vi "TTLConnect.vi"(0 "port":u16, 1 "error in":errorcluster) -> (2 "context out":refnum<class "zmq_context.lvclass">, 3 "socket out":refnum<class "zmq_socket.lvclass">, 4 "error out":errorcluster)   [LabVIEW 2017]
doc: "Opens a ZeroMQ socket and subscribes to OpenEphys TTL events."
uses:
  <vilib>/addons/zeromq/zmq_socket.lvclass
  <vilib>/addons/zeromq/zmq_context.lvclass
  <vilib>/addons/zeromq/socket_type.ctl
  <vilib>/addons/zeromq/socket_options.ctl
  EventBaseType.ctl
  <vilib>/addons/zeromq/zeromq.lvlib
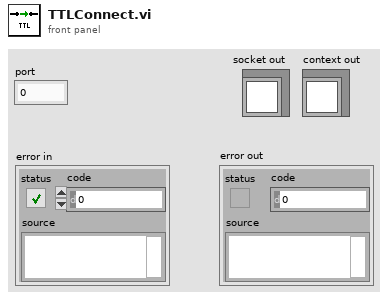
[diagram p1: front panel]
types:
  T1 = typedef "zeromq.lvlib/socket_options.ctl" = enum8{"NONE", "ZMQ_HWM", "<2>", "ZMQ_SWAP", "ZMQ_AFFINITY", "ZMQ_IDENTITY", "ZMQ_SUBSCRIBE", "ZMQ_UNSUBSCRIBE", "ZMQ_RATE", "ZMQ_RECOVERY_IVL", "ZMQ_MCAST_LOOP", "ZMQ_SNDBUF", "ZMQ_RCVBUF", "ZMQ_RCVMORE", "ZMQ_FD", "ZMQ_EVENTS", "ZMQ_TYPE", "ZMQ_LINGER", "ZMQ_RECONNECT_IVL", "ZMQ_BACKLOG", "ZMQ_RECOVERY_IVL_MSEC", "ZMQ_RECONNECT_IVL_MAX", "ZMQ_MAXMSGSIZE", "ZMQ_SNDHWM", "ZMQ_RCVHWM", "ZMQ_MULTICAST_HOPS", "<26>", "ZMQ_RCVTIMEO", "ZMQ_SNDTIMEO", "<29>", "<30>", "ZMQ_IPV4ONLY", "ZMQ_LAST_ENDPOINT", "ZMQ_ROUTER_MANDATORY", "ZMQ_TCP_KEEPALIVE", "ZMQ_TCP_KEEPALIVE_CNT", "ZMQ_TCP_KEEPALIVE_IDLE", "ZMQ_TCP_KEEPALIVE_INTVL", "ZMQ_TCP_ACCEPT_FILTER", "ZMQ_DELAY_ATTACH_ON_CONNECT", "ZMQ_XPUB_VERBOSE"}
  T2 = enum16{"big-endian, network order", "native, host order", "little-endian"}
  T3 = typedef "EventBaseType.ctl" = enum16{"SYSTEM_EVENT", "PROCESSOR_EVENT", "SPIKE_EVENT"}
  T4 = typedef "zeromq.lvlib/socket_type.ctl" = enum8{"ZMQ_PAIR", "ZMQ_PUB", "ZMQ_SUB", "ZMQ_REQ", "ZMQ_REP", "ZMQ_DEALER", "ZMQ_ROUTER", "ZMQ_PULL", "ZMQ_PUSH", "ZMQ_XPUB", "ZMQ_XSUB"}
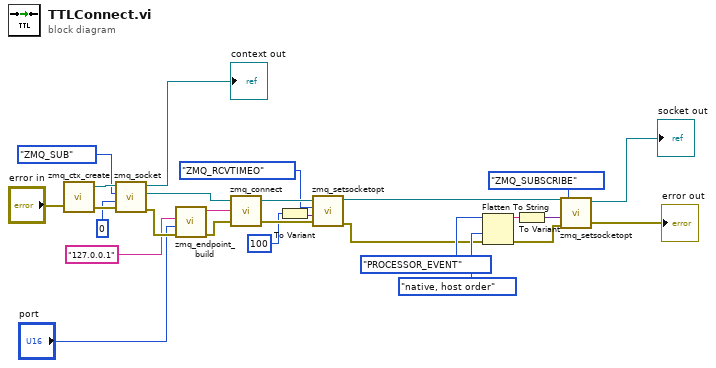
[diagram p0: block diagram]
diagram:
  n1 = call <vilib>:"zmq_ctx_create.vi"("error in"="error in") -> ("error out"=w27:errorcluster, "context out"=w26:refnum<class "zmq_context.lvclass">)  [unwired: 3 in]
  n2 = call <vilib>:"zmq_socket.vi"("error in"=w27, "linger (ms)"=0, "socket type"=socket_type."ZMQ_SUB", "context in"=w26) -> ("error out"=w18:errorcluster, "socket out"=w19:refnum<class "zmq_socket.lvclass">, "context out"=→"context out":refnum<class "zmq_context.lvclass">)  [unwired: 1 in]
  n3 = call <vilib>:"zmq_endpoint_build.vi"("error in"=w18, "port"="port", "address"="127.0.0.1" ("initial string")) -> ("error out"=w14:errorcluster, "endpoint"=w15:string)  [unwired: 2 in, 1 out]
  n4 = call <vilib>:"zmq_connect.vi"("error in"=w14, "endpoint"=w15, "socket in"=w19) -> ("error out"=w6:errorcluster, "socket out"=w7:refnum<class "zmq_socket.lvclass">)  [unwired: 1 in]
  n5 = To Variant(anything=100) -> (Variant=w2:variant)
  n6 = call <vilib>:"zmq_setsocketopt.vi"("error in"=w6, "value"=w2, "option"=socket_options."ZMQ_RCVTIMEO", "socket in"=w7) -> ("error out"=w5:errorcluster, "socket out"=w4:refnum<class "zmq_socket.lvclass">)  [unwired: 2 in]
  n7 = Flatten To String(anything=EventBaseType."PROCESSOR_EVENT", byte order (0:big-endian, network order)=T2."native, host order", error in (no error)=w5) -> (data string=w20:string, error out=w10:errorcluster)  [unwired: 1 in, 1 out]
  n8 = To Variant(anything=w20) -> (Variant=w21:variant)
  n9 = call <vilib>:"zmq_setsocketopt.vi"("error in"=w10, "value"=w21, "option"=socket_options."ZMQ_SUBSCRIBE", "socket in"=w4) -> ("error out"=→"error out":errorcluster, "socket out"=→"socket out":refnum<class "zmq_socket.lvclass">)  [unwired: 2 in]
